vi "First_QuVI_Wire.vi"(2 "QuVI in":refnum<class "QuSim.lvclass">[](array[class])) -> (8 "QuVI Wire out":refnum<class "QuWire.lvclass">, 13 "QuVI out":refnum<class "QuSim.lvclass">)   [LabVIEW 2020]
doc: "\"Initializes a qubit in the state |0> and provides a reference wire for circuit construction.\"\n\nThis VI serves as the fundamental starting point for any quantum circuit in the QuVI toolkit. It effectively initializes a single qubit in the ground state |0>.\n\nTo build a multi-qubit register, stack multiple instances of this VI vertically on the block diagram. The vertical connections aggregate the qubit count for the global state vector.\n\nTerminals:\n\n[Top] Stack In: Connect from the 'Stack Out' of the previous qubit above. Leave unconnected for the first qubit (Qubit 0).\n\n[Bottom] Stack Out: Connect to the 'Stack In' of the next qubit below.\n\n[Right] Quantum Wire Ref: The \"QuWire.\" Connect this to the left border of a Flat Sequence Structure."
uses:
  QuWire/QuWire.lvclass
  SimAlg/PrllPerElement/PrllPerElmnt.lvclass
  QuSim.lvclass
  SimAlg/QubitWise/QubitWiseMult.lvclass
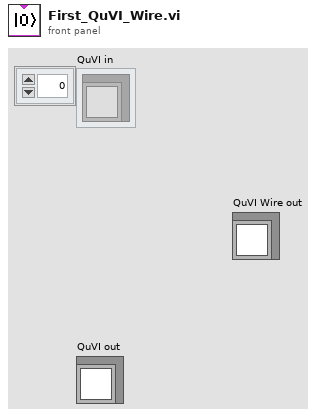
[diagram p1: front panel]
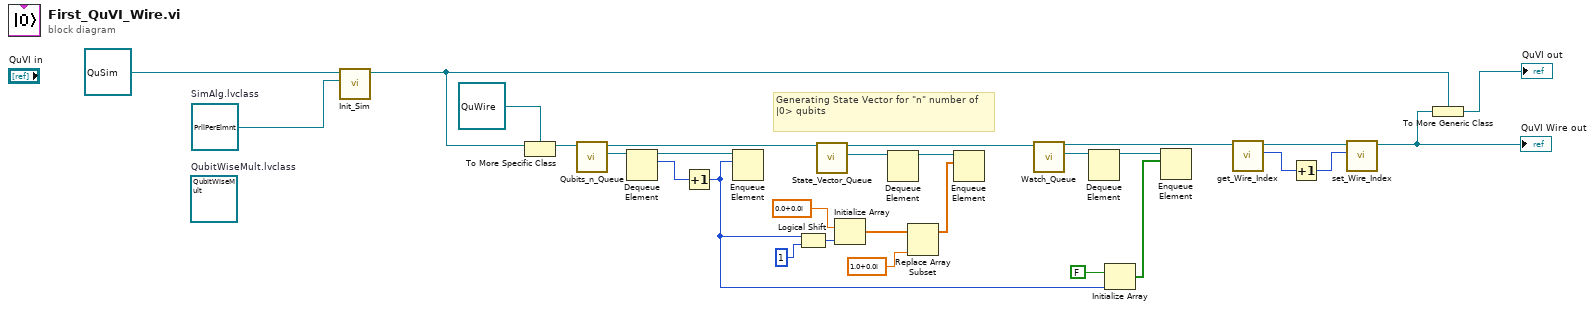
[diagram p0: block diagram]
diagram:
  (unwired) refnum<class "QubitWiseMult.lvclass"> refnum  # QubitWiseMult.lvclass
  w1 = refnum<class "PrllPerElmnt.lvclass"> refnum  # SimAlg.lvclass
  # "Generating State Vector for \"n\" number of |0> qubits"
  n1 = call "Init_Sim.vi"("SimAlg.lvclass"=w1, "QuSim in"=refnum<class "QuSim.lvclass"> refnum ("QuSim.lvclass")) -> ("QuSim out"=w3:refnum<class "QuSim.lvclass">)  [unwired: 9 in]
  n2 = To More Specific Class(target class=refnum<class "QuWire.lvclass"> refnum ("Wire.lvclass"), reference=w3) -> (specific class reference=w25:refnum<class "QuWire.lvclass">)  [unwired: 1 in, 1 out]
  n3 = call "Qubits_n_Queue.vi"("QuWire in"=w25) -> ("Qubit n"=w26:refnum<queue>, "QuWire out"=w8:refnum<class "QuWire.lvclass">)  [unwired: 8 in, 1 out]
  n4 = Dequeue Element(queue=w26) -> (queue out=w27:refnum<queue>, element=w28:i32)  [unwired: 2 in, 2 out]
  n5 = Increment(x=w28) -> (x+1=w9:i32)
  n6 = Enqueue Element(queue=w27, element=w9) -> ()  [unwired: 2 in, 3 out]
  n7 = Logical Shift(y=w9, x=u32 1) -> (x << y=w13:u32)
  n8 = call "State_Vector_Queue.vi"("QuWire in"=w8) -> ("State Vector Queue"=w16:refnum<queue>, "QuWire out"=w6:refnum<class "QuWire.lvclass">)  [unwired: 8 in, 1 out]
  n9 = Initialize Array(cdb 0.0+0.0i ("element"), w13) -> (w12:cdb[])
  n10 = Dequeue Element(queue=w16) -> (queue out=w17:refnum<queue>)  [unwired: 2 in, 3 out]
  n11 = Replace Array Subset(array=w12, new element=cdb 1.0+0.0i ("element")) -> (w10:cdb[])  [unwired: 1 in]
  n12 = Enqueue Element(queue=w17, element=w10) -> ()  [unwired: 2 in, 3 out]
  n13 = call "Watch_Queue.vi"("QuWire in"=w6) -> ("Watch List"=w19:refnum<queue>, "QuWire out"=w7:refnum<class "QuWire.lvclass">)  [unwired: 8 in, 1 out]
  n14 = Dequeue Element(queue=w19) -> (queue out=w20:refnum<queue>)  [unwired: 2 in, 3 out]
  n15 = Initialize Array(FALSE, w9) -> (w21:bool[])
  n16 = Enqueue Element(queue=w20, element=w21) -> ()  [unwired: 2 in, 3 out]
  n17 = call "get_Wire_Index.vi"("QuWire in"=w7) -> ("Wire Index"=w23:i32, "QuWire out"=w22:refnum<class "QuWire.lvclass">)  [unwired: 8 in, 1 out]
  n18 = Increment(x=w23) -> (x+1=w24:i32)
  n19 = call "set_Wire_Index.vi"("Wire Index"=w24, "QuWire in"=w22) -> ("QuWire out"=w5:refnum<class "QuWire.lvclass">)  [unwired: 8 in, 1 out]
  "QuVI Wire out" <- w5
  n20 = To More Generic Class(target class=w3, reference=w5) -> (generic class reference=→"QuVI out":refnum<class "QuSim.lvclass">)
